vi "Create Server.vi"(8 "error in":errorcluster) -> (0 "error out":errorcluster, 3 "gRPCid out":T1)   [LabVIEW 2019, in "grpc-lvsupport.lvlib"]
uses:
  grpc-lvsupport.lvlib
  grpcId.ctl
  <vilib>/Utility/file.llb/Application Directory.vi
  <vilib>/Utility/error.llb/Error Cluster From Error Code.vi
  <resource>/labview_grpc_server.dll
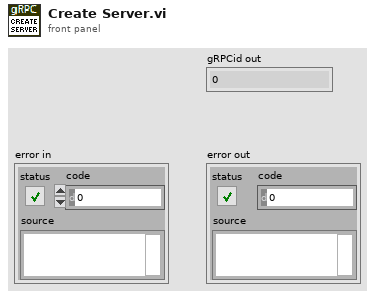
[diagram p1: front panel]
types:
  T1 = typedef "grpc-lvsupport.lvlib/grpcId.ctl" = u64
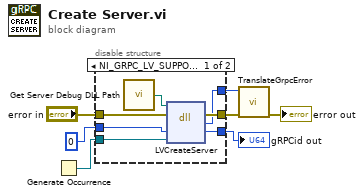
[diagram p0: block diagram]
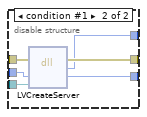
[diagram p2: hidden frame]
diagram:
  n1 = Generate Occurrence() -> (w2:refnum<k4>)
  n2 = disable-structure shown="NI_GRPC_LV_SUPPORT_DEBUG==True&&RUN_TIME_ENGINE==False" {
    disable-tunnel: "error in" -> [w14 w20]
    disable-tunnel: [w13 w19] -> w3
    disable-tunnel: [w12 w18] -> w7
    disable-tunnel: [w10 w17] -> w5
    disable-tunnel: w2 -> [w9 w16]
    disable-tunnel: u64 0 ("server") -> [w8 w15]
    frame condition #0 (active) {
      n3 = call "Get Server Debug DLL Path.vi"() -> ("DLL Path"=w11:path)
      n4 = dll-call lib="?" fn="LVCreateServer"(path in=w11, error in=w14, "server"=w8, "InitCallbackOccurrence"=w9) -> (error out=w13:errorcluster, "return type"=w10:i32, "server"=w12:u64)  [unwired: 2 in, 1 out]
    }
    frame condition #1 {
      n5 = dll-call lib="C:/Program Files (x86)/National Instruments/LabVIEW 2024/resource/labview_grpc_server.*" fn="LVCreateServer"(error in=w20, "server"=w15, "InitCallbackOccurrence"=w16) -> (error out=w19:errorcluster, "return type"=w17:i32, "server"=w18:u64)  [unwired: 3 in, 1 out]
    }
  }
  "gRPCid out" <- w7
  n6 = call "TranslateGrpcError.vi"("error in"=w3, "Error Code"=w5) -> ("error out"=→"error out":errorcluster)  [unwired: 9 in]
